vi "Library Check Path.vi"(4 "error in (no error)":errorcluster, 5 "directory (true)":bool=TRUE, 6 "further explanation (none)":string, 7 "path":path) -> (0 "error out":errorcluster, 3 "dup path":path)   [LabVIEW 2012]
doc: "Check a path. This VI throws a readable error when the expected file or directory does not exist."
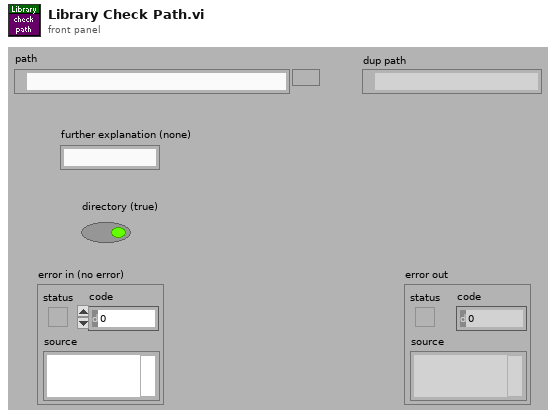
[diagram p1: front panel]
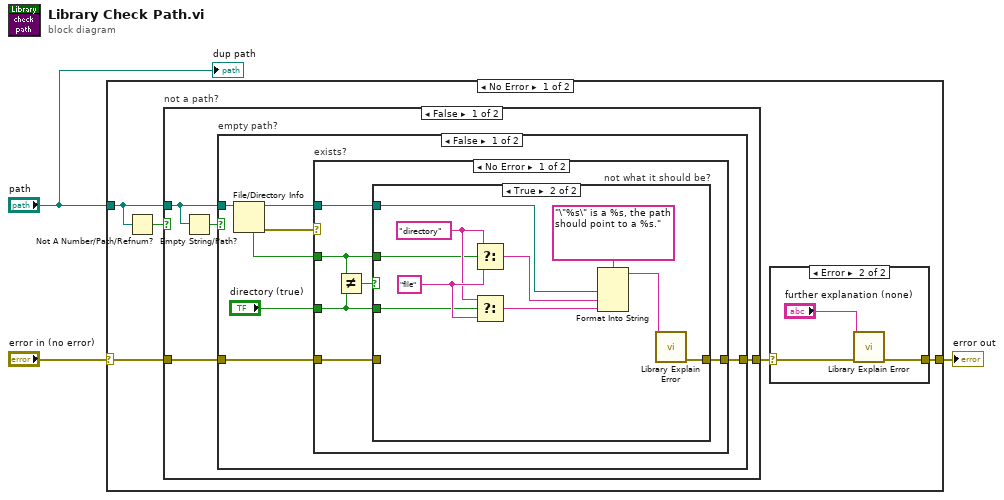
[diagram p0: block diagram]
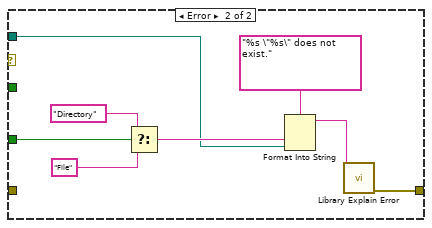
[diagram p3: hidden frame]
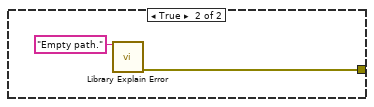
[diagram p4: hidden frame]
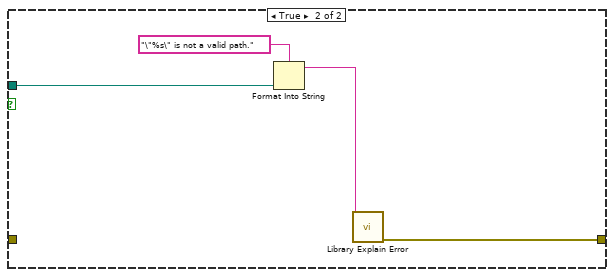
[diagram p5: hidden frame]
diagram:
  n1 = case shown="No Error" "error in (no error)" {
    selector: "error in (no error)" -> [w8 w55]
    tunnel: [w6 w55] -> w3
    tunnel: "path" -> [w5 _]
    frame No Error {
      n2 = Not A Number/Path/Refnum?(number/path/refnum=w5) -> (NaN/Path/Refnum?=w4:bool)
      n3 = case "not a path?" shown="False" w4 {
        tunnel: w8 -> [w12 _]
        tunnel: [w11 w50] -> w7
        tunnel: w5 -> [w9 w49]
        frame False {
          n4 = Empty String/Path?(string/path=w9) -> (empty?=w10:bool)
          n5 = case "empty path?" shown="False" w10 {
            tunnel: w9 -> [w19 _]
            tunnel: w12 -> [w17 _]
            tunnel: [w14 w46] -> w11
            frame False {
              n6 = File/Directory Info(path=w19) -> (path out=w18:path, directory=w13:bool, error out=w16:errorcluster)  [unwired: 1 in, 4 out]
              n7 = case "exists?" shown="No Error" w16 {
                tunnel: [w23 w44] -> w14
                tunnel: w18 -> [w22 w37]
                tunnel: w17 -> [w24 _]
                tunnel: "directory (true)" -> [w21 w41]
                tunnel: w13 -> [w20 _]
                frame No Error {
                  n8 = Not Equal?(x=w20, y=w21) -> (x != y?=w25:bool)
                  n9 = case "not what it should be?" shown="True" w25 {
                    tunnel: w24 -> [w26 _]
                    tunnel: [w26 w28] -> w23
                    tunnel: w22 -> [_ w33]
                    tunnel: w21 -> [_ w31]
                    tunnel: w20 -> [_ w32]
                    frame False {
                    }
                    frame True {
                      w36 = "file"
                      w35 = "directory"
                      n10 = Select(t=w35, s=w32, f=w36) -> (s? t:f=w30:string)
                      n11 = Select(t=w35, s=w31, f=w36) -> (s? t:f=w29:string)
                      n12 = Format Into String(format string="\"%s\" is a %s, the path should point to a %s.", w33, w30, w29) -> (resulting string=w27:string)  [unwired: 2 in, 1 out]
                      n13 = call "Library Explain Error.vi"("explanation prefix (none)"=w27) -> ("explained error"=w28:errorcluster)  [unwired: 14 in]
                    }
                  }
                }
                frame Error {
                  n14 = Select(t="Directory", s=w41, f="File") -> (s? t:f=w38:string)
                  n15 = Format Into String(format string="%s \"%s\" does not exist.", w38, w37) -> (resulting string=w42:string)  [unwired: 2 in, 1 out]
                  n16 = call "Library Explain Error.vi"("explanation prefix (none)"=w42) -> ("explained error"=w44:errorcluster)  [unwired: 14 in]
                }
              }
            }
            frame True {
              n17 = call "Library Explain Error.vi"("explanation prefix (none)"="Empty path.") -> ("explained error"=w46:errorcluster)  [unwired: 14 in]
            }
          }
        }
        frame True {
          n18 = Format Into String(format string="\"%s\" is not a valid path.", w49) -> (resulting string=w48:string)  [unwired: 2 in, 1 out]
          n19 = call "Library Explain Error.vi"("explanation prefix (none)"=w48) -> ("explained error"=w50:errorcluster)  [unwired: 14 in]
        }
      }
      n20 = case shown="Error" w7 {
        selector: w7 -> [w51 w54]
        tunnel: [w51 w52] -> w6
        frame No Error {
        }
        frame Error {
          n21 = call "Library Explain Error.vi"("explanation prefix (none)"="further explanation (none)", "error in (no error)"=w54) -> ("explained error"=w52:errorcluster)  [unwired: 13 in]
        }
      }
    }
    frame Error {
    }
  }
  "error out" <- w3
  "dup path" <- "path"
